vi "SpectraPro-open.vi"(5 "VISA resource name":refnum<visa-resource-name>="COM12") -> (0 "error out":errorcluster, 1 "status":bool=TRUE, 2 "VISA resource name out":refnum<visa-resource-name>)   [LabVIEW 2014]
doc: "Andre Romero - 2016\nandretec@ifsc.usp.br\nIFSC - USP"
uses:
  <vilib>/Instr/_visa.llb/VISA Configure Serial Port (Instr).vi
panel:
  out "bytes read":u32=233
  out "read string":string="\r\nINITIALIZING\r\nActon Research Corp.  SP-150  V1.4  \r\n?NM 435.8  ok\r\n?NM 435.8  ok\r\n?NM 435.8  ok\r\n?NM 435.8  ok\r\n?NM 435.8  ok\r\n?NM 435.8  ok\r\n?NM 435.8  ok\r\n?NM 435.8  ok\r\n?NM 435.8  ok\r\n?NM 435.8  ok\r\n?NM 435.8  ok\r\n?NM 435.8  ok\r\n?NM 435.8  ok\r\n"
  # "0 - Select the Com Port Number\n1 - RUN the program\n2 - Turn on the Power Supply of the Spectrometer\n3 - Whait for the Initialization ......"
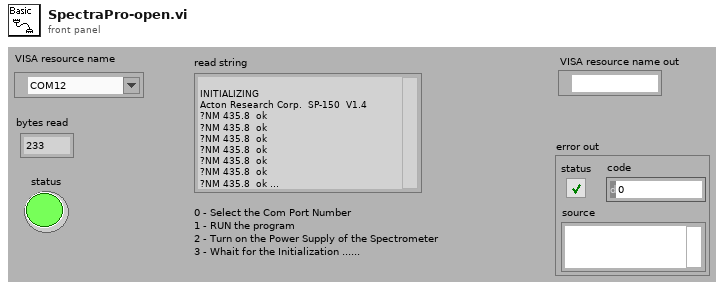
[diagram p1: front panel]
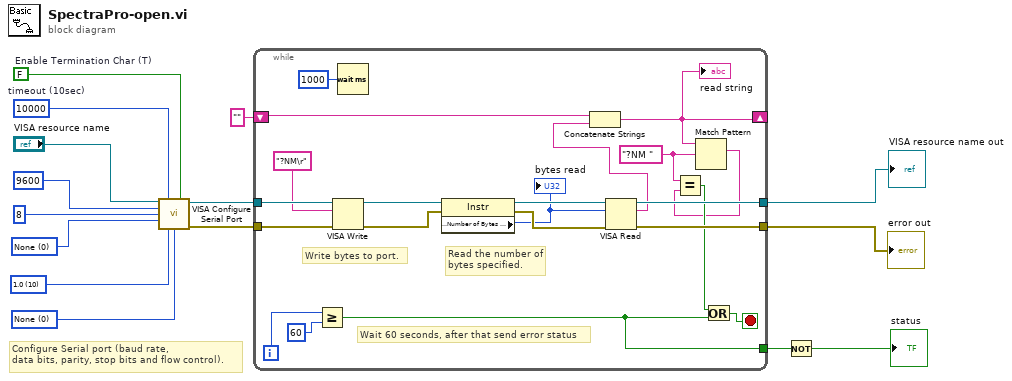
[diagram p0: block diagram]
diagram:
  w7 = u16 0 items=["None"=0, "XON/XOFF"=1, "RTS/CTS"=2, "DTR/DSR"=4] ("flow control")
  w8 = u16 10 items=["1.0"=10, "1.5"=15, "2.0"=20] ("stop bits")
  w11 = u16 0 items=["None", "Odd", "Even", "Mark", "Space"] ("parity")
  w9 = FALSE  # Enable Termination Char (T)
  w10 = u32 10000  # timeout (10sec)
  # "Configure Serial port (baud rate,\ndata bits, parity, stop bits and flow control)."
  n1 = call-poly "VISA Configure Serial Port"("VISA resource name"="VISA resource name", "timeout (10sec)"=w10, "Enable Termination\nChar (T)"=w9, "baud rate (9600)"=u32 9600 ("baud rate"), "data bits (8)"=u16 8 ("data bits"), "parity (0:none)"=w11, "stop bits (10: 1 bit)"=w8, "flow control (0:none)"=w7) -> ("VISA resource name out"=w12:refnum<visa-resource-name>, "error out"=w13:errorcluster)  [unwired: 6 in]
  n2 = while {
    tunnel: w13 -> [w36]
    tunnel: w12 -> [w35]
    tunnel: [w34] -> w3
    tunnel: [w33] -> w4
    shift-right: [w23] -> _
    shift-left: "" -> [w26]
    tunnel: [w17] -> w2
    i -> [w20]
    stop <- w18 stop-if-true
    w24 = "?NM " ("regular expression")
    # "Wait 60 seconds, after that send error status"
    # "Read the number of bytes specified."
    # "Write bytes to port."
    n3 = Greater Or Equal?(x=w20, y=60) -> (x >= y?=w17:bool)
    n4 = VISA Write(VISA resource name=w35, write buffer="?NM\r" ("string to write"), error in (no error)=w36) -> (VISA resource name out=w31:refnum<visa-resource-name>, error out=w32:errorcluster)  [unwired: 1 out]
    n5 = Wait (ms)(milliseconds to wait=u32 1000) -> ()  [unwired: 1 out]
    n6 = property class="Instr"(reference=w31, error in=w32) -> (reference out=w29:refnum<visa-resource-name>, error out=w28:errorcluster, "Serial Settings:Number of Bytes at Serial Port"=w27:u32)
    "bytes read" <- w27
    n7 = VISA Read(VISA resource name=w29, byte count=w27, error in (no error)=w28) -> (VISA resource name out=w33:refnum<visa-resource-name>, read buffer=w25:string, error out=w34:errorcluster)  [unwired: 1 out]
    n8 = Concatenate Strings(w26, w25) -> (w23:string)
    "read string" <- w23
    n9 = Match Pattern(string=w23, regular expression=w24) -> (match substring=w16:string)  [unwired: 1 in, 3 out]
    n10 = Equal?(x=w24, y=w16) -> (x = y?=w21:bool)
    n11 = Or(x=w21, y=w17) -> (x .or. y?=w18:bool)
  }
  "VISA resource name out" <- w4
  "error out" <- w3
  n12 = Not(x=w2) -> (.not. x?=→"status":bool)
